vi "Tosca-Check For Output Parser End.vi"(0 "Parse End Queue In":refnum<queue>, 7 "State":i32, 9 "AO in":dbl[][](array[numeric]), 11 "error in (no error)":errorcluster, 13 "ramp off":bool[](array[boolean])) -> (4 "Parse End Queue Out":refnum<queue>, 6 "End?":bool, 10 "AO out":dbl[][](array[numeric]), 15 "error out":errorcluster)   [LabVIEW 2020]
uses:
  Typedefs/Tosca-End Parser Queue Data.ctl
  Trace VIs/Tosca-Trace-Event.ctl
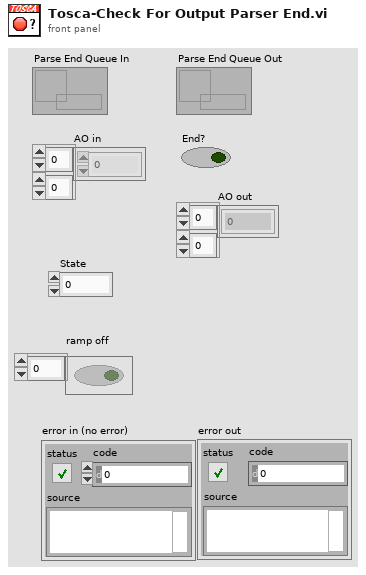
[diagram p1: front panel]
types:
  T1 = typedef "Tosca-End Parser Queue Data.ctl" = cluster{"Quit":bool, "State":i32}
  T2 = typedef "Tosca-Trace-Event.ctl" = enum16{"Unspecified", "Trial start", "Enqueue", "Result", "End parser", "Frame", "Queue available", "Timeout sent", "WritePos", "TTL"}
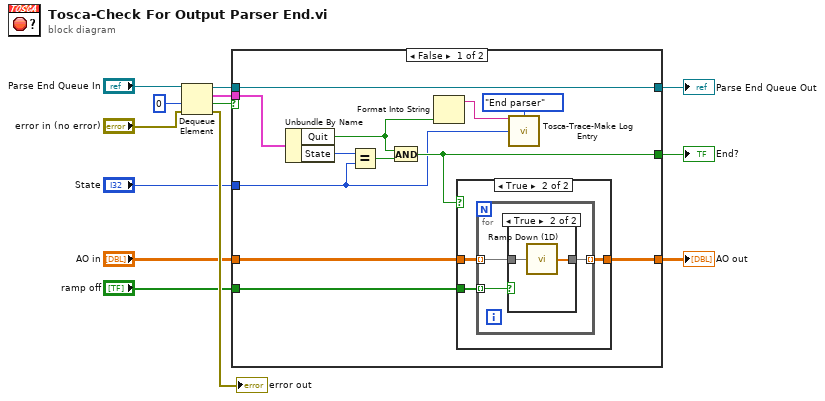
[diagram p0: block diagram]
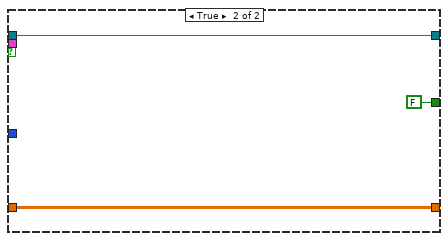
[diagram p4: hidden frame]
diagram:
  n1 = Dequeue Element(queue="Parse End Queue In", timeout in ms (-1)=0, error in (no error)="error in (no error)") -> (queue out=w4:refnum<queue>, element=w6:T1, timed out?=w2:bool, error out=→"error out":errorcluster)
  n2 = case shown="False" w2 {
    tunnel: [w25 FALSE] -> w12
    tunnel: [w18 w37] -> w10
    tunnel: "AO in" -> [w17 w37]
    tunnel: "State" -> [w14 _]
    tunnel: "ramp off" -> [w24 _]
    tunnel: w6 -> [w23 _]
    tunnel: w4 -> [w19 w36]
    tunnel: [w19 w36] -> w3
    frame False {
      n3 = Unbundle By Name(w23) -> ("Quit"=w16:bool, "State"=w22:i32)
      n4 = Equal?(x=w22, y=w14) -> (x = y?=w21:bool)
      n5 = And(x=w16, y=w21) -> (x .and. y?=w25:bool)
      n6 = Format Into String(w16) -> (resulting string=w15:string)  [unwired: 3 in, 1 out]
      n7 = case shown="True" w25 {
        tunnel: w17 -> [w26 w29]
        tunnel: [w26 w27] -> w18
        tunnel: w24 -> [_ w28]
        frame False {
        }
        frame True {
          n8 = for {
            tunnel: w29 -> [w31] mode=indexing
            tunnel: w28 -> [w32] mode=indexing
            tunnel: [w30] -> w27 mode=indexing
            n9 = case shown="True" w32 {
              tunnel: w31 -> [w33 w35]
              tunnel: [w33 w34] -> w30
              frame False {
              }
              frame True {
                n10 = call "Ramp Down (1D).vi"("Array"=w35) -> ("Ramped array"=w34:dbl[])  [unwired: 4 in]
              }
            }
          }
        }
      }
      n11 = call "Tosca-Trace-Make Log Entry.vi"("Message"=w15, "Event"=Tosca-Trace-Event."End parser", "Value"=w14) -> ()  [unwired: 12 in, 1 out]
    }
    frame True {
    }
  }
  "Parse End Queue Out" <- w3
  "End?" <- w12
  "AO out" <- w10
